vi "Default Instrument Setup.vi"(7 "Channel (0: Channel A)":u16(ring) items=["Channel A", "Channel B"], 8 "error in (no error)":errorcluster, 11 "BH Druck PACE Series in":refnum<class "BH Druck PACE Series.lvclass">) -> (0 "error out":errorcluster, 3 "BH Druck PACE Series out":refnum<class "BH Druck PACE Series.lvclass">)   [LabVIEW 2022 SP3, in "BH Druck PACE Series.lvclass"]
uses:
  BH Druck PACE Series.lvclass
  BH Druck PACE Series.lvclass/BH Druck PACE Series.ctl
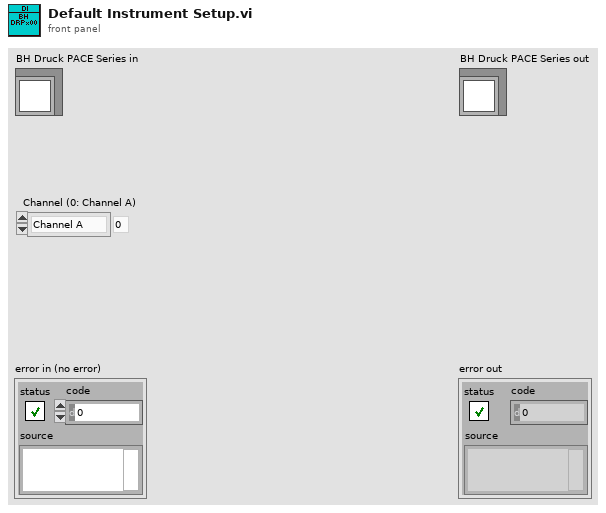
[diagram p1: front panel]
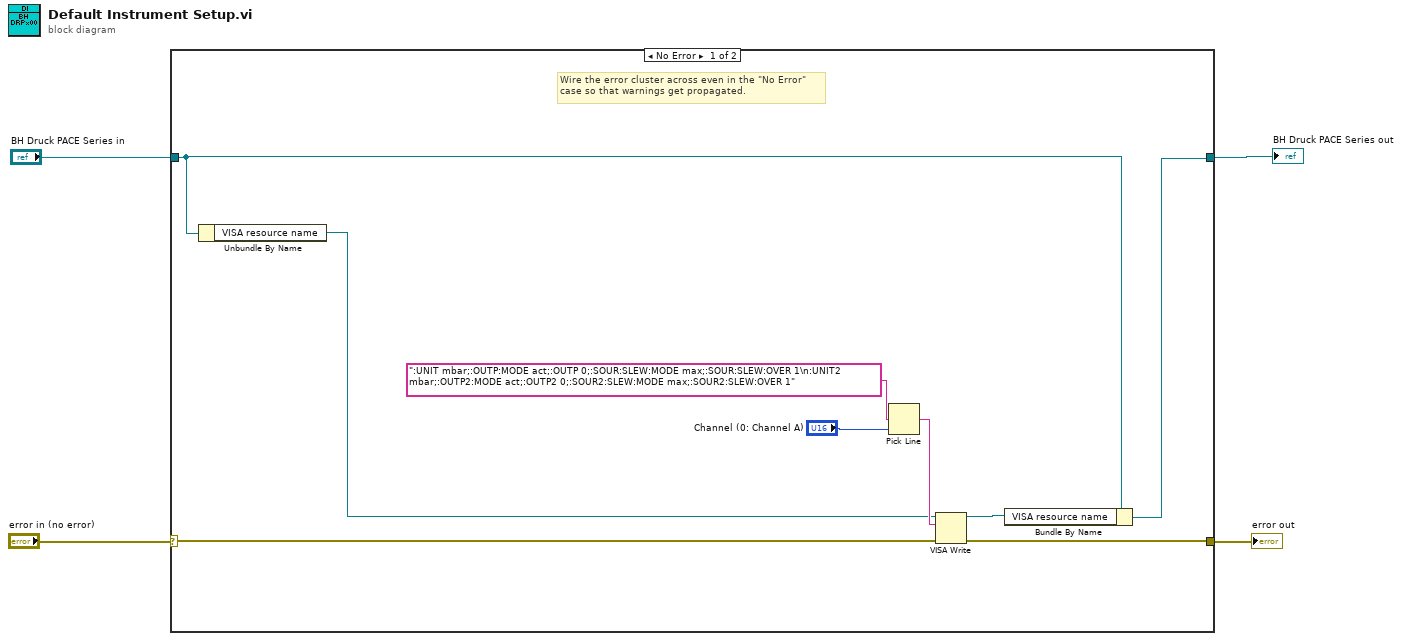
[diagram p0: block diagram]
diagram:
  n1 = case shown="No Error" "error in (no error)" {
    selector: "error in (no error)" -> [w10 w15]
    tunnel: [w8 w15] -> w3
    tunnel: [w5 w14] -> w1
    tunnel: "BH Druck PACE Series in" -> [w7 w14]
    frame No Error {
      # "Wire the error cluster across even in the \"No Error\"\ncase so that warnings get propagated."
      n2 = Unbundle By Name(w7) -> ("VISA resource name"=w9:refnum<visa-resource-name>)
      n3 = Pick Line(multi-line string=":UNIT mbar;:OUTP:MODE act;:OUTP 0;:SOUR:SLEW:MODE max;:SOUR:SLEW:OVER 1\n:UNIT2 mbar;:OUTP2:MODE act;:OUTP2 0;:SOUR2:SLEW:MODE max;:SOUR2:SLEW:OVER 1", line index="Channel (0: Channel A)") -> (output string=w13:string)  [unwired: 1 in]
      n4 = VISA Write(VISA resource name=w9, write buffer=w13, error in (no error)=w10) -> (VISA resource name out=w6:refnum<visa-resource-name>, error out=w8:errorcluster)  [unwired: 1 out]
      n5 = Bundle By Name(cluster=w7, "VISA resource name"=w6) -> (w5:refnum<class "BH Druck PACE Series.lvclass">)
    }
    frame Error {
    }
  }
  "error out" <- w3
  "BH Druck PACE Series out" <- w1
